vi "SMTP Email Close Session.vi"(4 "error in (no error)":errorcluster, 7 "smtp session":T1) -> (0 "error out":errorcluster, 3 "smtp session out":T1)   [LabVIEW 2011, in "NewNI_SMTPEmail.lvlib"]
doc: "This VI sends the QUIT command to the SMTP server, and then closes TCP connection specified as \"Connection ID\". It propagates any error occured in (or before) the call to this VI through the \"error out\" cluster."
uses:
  NewNI_SMTPEmail.lvlib
  SMTP Email Session.ctl
panel:
  in  "tcp connection":refnum<k5>
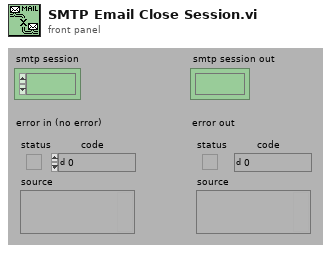
[diagram p1: front panel]
types:
  T1 = typedef "NewNI_SMTPEmail.lvlib/SMTP Email Session.ctl" = refnum<k1>
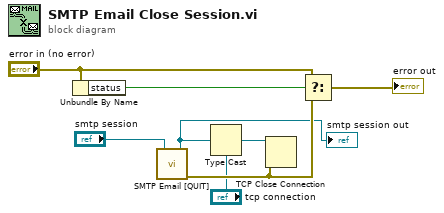
[diagram p0: block diagram]
diagram:
  n1 = Unbundle By Name("error in (no error)") -> ("status"=w8:bool)
  n2 = call "SMTP Email [QUIT].vi"("smtp session"="smtp session") -> ("error out"=w5:errorcluster, "smtp session out"=w4:T1)  [unwired: 2 in, 3 out]
  "smtp session out" <- w4
  n3 = Type Cast(type="tcp connection", x=w4) -> (*(type *) &x=w3:refnum<k5>)
  n4 = TCP Close Connection(connection ID=w3, error in (no error)=w5) -> ()  [unwired: 3 out]
  n5 = Select(t="error in (no error)", s=w8, f=w5) -> (s? t:f=→"error out":errorcluster)
